vi "Add to Type Descriptor Map.vi"(8 "error in (no error)":errorcluster, 9 "Type Descriptor":i16[](array[numeric]), 10 "Type Name":string, 11 "TwinCAT ADS in":refnum<class "TwinCAT ADS.lvclass">) -> (0 "error out":errorcluster, 1 "Replaced?":bool, 3 "TwinCAT ADS out":refnum<class "TwinCAT ADS.lvclass">)   [LabVIEW 2018, in "TwinCAT ADS.lvclass"]
uses:
  TwinCAT ADS.lvclass
  TwinCAT ADS.lvclass/TwinCAT ADS.ctl
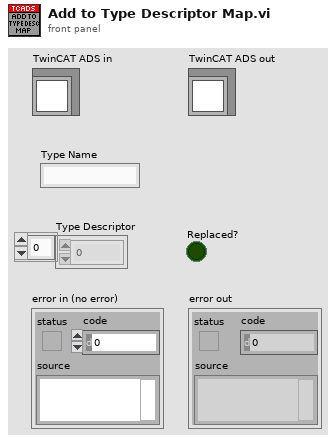
[diagram p1: front panel]
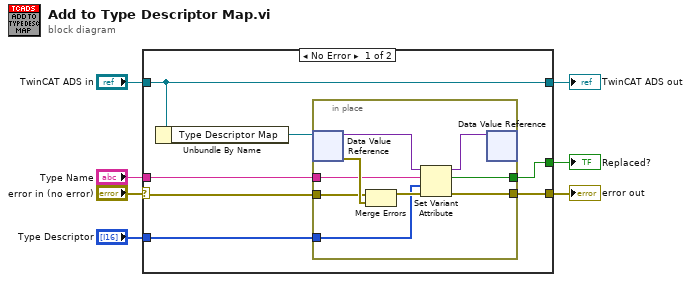
[diagram p0: block diagram]
diagram:
  n1 = case shown="No Error" "error in (no error)" {
    selector: "error in (no error)" -> [w9 w25]
    tunnel: [w11 w25] -> w6
    tunnel: [w13 w24] -> w4
    tunnel: "TwinCAT ADS in" -> [w13 w24]
    tunnel: "Type Descriptor" -> [w12 _]
    tunnel: [w10 _] -> w2
    tunnel: "Type Name" -> [w8 _]
    frame No Error {
      n2 = Unbundle By Name(w13) -> ("Type Descriptor Map"=w14:refnum<data-value>)
      n3 = in-place {
        in-place-border: w9 -> [w19]
        in-place-border: w8 -> [w20]
        in-place-border: w12 -> [w17]
        in-place-border: [w16] -> w11
        in-place-border: [w15] -> w10
        n4 = in-place-dvr #1(w14) -> (w22:variant, w23:errorcluster)
        n5 = Merge Errors(w19, w23) -> (w18:errorcluster)
        n6 = Set Variant Attribute(Variant=w22, name=w20, value=w17, error in=w18) -> (Variant out=w21:variant, replaced=w15:bool, error out=w16:errorcluster)
        n7 = in-place-dvr #1(w21) -> ()  [unwired: 2 out]
      }
    }
    frame Error {
    }
  }
  "error out" <- w6
  "TwinCAT ADS out" <- w4
  "Replaced?" <- w2
